vi "Write Cap to sweep.vi"(10 "Cap to sweep":T1[](array[typedef]), 11 "Toggle 6 in":refnum<class "Toggle 7.1.lvclass">) -> (3 "Toggle 6 out":refnum<class "Toggle 7.1.lvclass">)   [LabVIEW 2020, in "Toggle 7.1.lvclass"]
uses:
  Toggle 7.1.lvclass
  Controls/Parameter Cluster.ctl
  Toggle 7.1.lvclass/Toggle 7.1.ctl
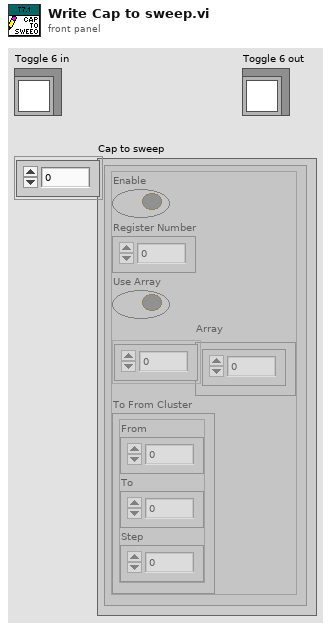
[diagram p1: front panel]
types:
  T1 = typedef "Toggle 7.1.lvclass/Parameter Cluster.ctl" = cluster{"Enable":bool, "Register Number":u32, "Use Array":bool, "Array":dbl[], "To From Cluster":cluster{"From":dbl, "To":dbl, "Step":dbl}}
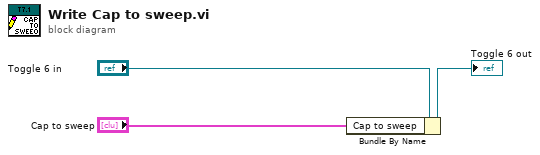
[diagram p0: block diagram]
diagram:
  n1 = Bundle By Name(cluster="Toggle 6 in", "Cap to sweep"="Cap to sweep") -> (→"Toggle 6 out":refnum<class "Toggle 7.1.lvclass">)
